vi "Append Table.vi"(0 "PDF Report IN":T30(xcontrol), 1 "Title format":T2={"Font"={"Name"="", "Size"=-1.0, "Color"=0, "Style"={"Bold"=TRUE, "Italic"=FALSE, "Underline"=FALSE, "Strikeout"=FALSE}}, "Align. and LS"={"Horizontal"=enum."CENTER", "Vertical"=enum."MIDDLE", "Line spacing"=enum."1.0"}}, 2 "Predefined Borders":T14={"Borders"=1, "Title"={"Thickness"=1.0, "Line"=0, "Background "=16777215}, "Datas"={"Thickness"=0.5, "Line"=0, "Background "=16777215}}, 3 "Row background color":T9={"color"=16777225, "at each"=0.0}, 7 "PDF Table":T1(xcontrol), 9 "Caption":string, 11 "error in (no error)":errorcluster, 12 "Datas format":T2={"Font"={"Name"="", "Size"=-1.0, "Color"=0, "Style"={"Bold"=FALSE, "Italic"=FALSE, "Underline"=FALSE, "Strikeout"=FALSE}}, "Align. and LS"={"Horizontal"=enum."CENTER", "Vertical"=enum."MIDDLE", "Line spacing"=enum."1.0"}}, 13 "Custom Borders":T13={"Title Row Border"={"Line"={"Thickness"=1.0, "Color"=0}, "Column Borders [ ]"=[]}, "Datas Row Borders [ ]"=[]}) -> (4 "PDF Report OUT":T30(xcontrol), 15 "error out":errorcluster)   [LabVIEW 2012]
doc: "<B>ENGLISH</B>\nAppends a table to the PDF document.\n\n<B>FRANÇAIS</B>\nAjoute un tableau au document PDF.\n\nDeveloped by Jean-Marc Simard\nCopyright © 2010, Exaprom Inc.\nAll rights reserved.\nLicense: BSD\n\nWith iTextSharp 4.1.6 (http://itextsharp.sourceforge.net)\nunder Mozilla Public License Version 1.1\n(http://www.mozilla.org/MPL/MPL-1.1.html)"
uses:
  Controls/PDF Report Xcontrol/PDF Report.xctl
  Controls/Row Predefined borders cluster.ctl
  Controls/Row Predefined borders.ctl
  Controls/Row Border Title.ctl
  Controls/Cell Border.ctl
  Controls/Row Borders [ ] Datas.ctl
  Controls/Row Back Ground color Datas.ctl
  Controls/Cell Properties Table.ctl
  Controls/Font cluster.ctl
  Controls/Font size.ctl
  Controls/Font color.ctl
  Controls/Texte alignement.ctl
  Controls/Cell Vertical alignment.ctl
  Controls/Line spacing.ctl
  Controls/PDF Table Xcontrol/PDF Table XControl.xctl
  Controls/Row borders from.ctl
  C:/Users/MaxCorp/Documents/TopPerm - Base/DLL/itextsharp.dll
  DLL/itextsharp.dll
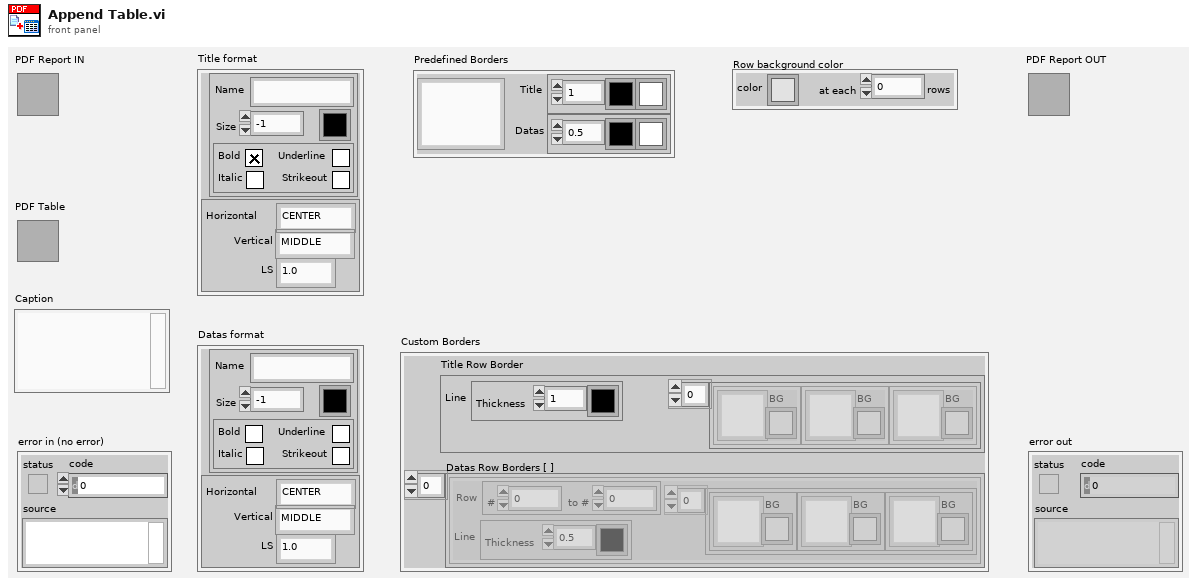
[diagram p1: front panel]
types:
  T1 = cluster{"PDFTable ref":refnum<k24>, "columnWidth (points)":sgl[], "Title 1D":string[], "Table Datas 2D":string[][], "Image to Add with refnum[ ]":cluster{"Image name":string, "InstanceImage":refnum<k24>}[]}
  T2 = typedef "Cell Properties Table.ctl" = cluster{"Font":T3, "Align. and LS":cluster{"Horizontal":T6, "Vertical":T7, "Line spacing":T8}}
  T3 = typedef "Font cluster.ctl" = cluster{"Name":string, "Size":T4, "Color":T5, "Style":cluster{"Bold":bool, "Italic":bool, "Underline":bool, "Strikeout":bool}}
  T4 = typedef "Font size.ctl" = sgl
  T5 = typedef "Font color.ctl" = u32
  T6 = typedef "Texte alignement.ctl" = enum16{"Select", "CENTER", "JUSTIFY", "LEFT", "RIGHT"}
  T7 = typedef "Cell Vertical alignment.ctl" = enum16{"TOP", "MIDDLE", "BOTTOM"}
  T8 = typedef "Line spacing.ctl" = enum16{"Select", "1.0", "1.5", "2.0"}
  T9 = typedef "Row Back Ground color Datas.ctl" = cluster{"color":u32, "at each":dbl}
  T10 = typedef "Row Border Title.ctl" = cluster{"Line":cluster{"Thickness":sgl, "Color":u32}, "Column Borders [ ]":cluster{"Cell Border":T11, "BG":u32}[]}
  T11 = typedef "Cell Border.ctl" = u16
  T12 = typedef "Row Borders [ ] Datas.ctl" = cluster{"Row":cluster{"#":i16, "to #":i16}, "Line":cluster{"Thickness":sgl, "Color":u32}, "Column Borders [ ]":cluster{"Cell Border":T11, "BG":u32}[]}[]
  T13 = cluster{"Title Row Border":T10, "Datas Row Borders [ ]":T12}
  T14 = typedef "Row Predefined borders cluster.ctl" = cluster{"Borders":T15, "Title":cluster{"Thickness":sgl, "Line":u32, "Background ":u32}, "Datas":cluster{"Thickness":sgl, "Line":u32, "Background ":u32}}
  T15 = typedef "Row Predefined borders.ctl" = u16
  T16 = typedef "Unit.ctl" = enum16{"inch", "mm"}
  T17 = typedef "Paragraphe cluster.ctl" = cluster{" Aligment":T6, "Line spacing":T8}
  T18 = typedef "Page dimensions.ctl" = cluster{"Start at page":i32, "Orientation":T19, "widht":sgl, "height":sgl, "Margin left":sgl, "Margin right":sgl, "Margin top":sgl, "Margin bottom":sgl}
  T19 = typedef "Page Orientation.ctl" = enum16{"Portrait", "Landscape"}
  T20 = typedef "Image or Table Caption.ctl" = cluster{"Caption":string, "Separator":string, "Position":enum16{"Above", "Below"}}
  T21 = typedef "Header Footer [ ].ctl" = T22[]
  T22 = typedef "Header Footer cluster.ctl" = cluster{"Start page":i32, "Type":T23, "Alignment":T24, "Vertical Alignement":T7, "Image (%)":sgl, "Page #":T25, "Text":string, "Path":string, "Font":T3, "Font refnum":refnum<k24>, "Line":cluster{"Line":T26, "Thickness (points)":sgl, "Colour":T5}}
  T23 = typedef "Header Footer Type.ctl" = enum16{"Select", "Text", "Text + hyperlink", "Page number", "Image", "Image + hyperlink"}
  T24 = typedef "Header footer horiz alignment.ctl" = enum16{"Left", "Center", "Right"}
  T25 = typedef "Page number.ctl" = cluster{"Text 1":string, "Text 2":string, "Text 3":string}
  T26 = typedef "Header Footer Line.ctl" = enum16{"No line", "Horizontal line"}
  T27 = typedef "Watermark cluster2.ctl" = cluster{"Show? (F)":bool, "Type":enum16{"Image", "Text"}, "Opacity (%)":sgl, "Rotate(°)":sgl, "Position":cluster{"Position":T28, "X":sgl, "Y":sgl}, "Image path":path, "Scaled(%)":sgl, "Image refnum":refnum<k24>, "Text":string, "Font":cluster{"Name":string, "Size":T4, "Color":T5}, "Font refnum":refnum<k24>, "Alignment":T24, "Automatic":bool}
  T28 = typedef "Watermark Position.ctl" = enum16{"Absolute", "Center (page)", "Center (text section)"}
  T29 = typedef "System Fonts.ctl" = cluster{"Font name [ ]":string[], "Font and file names [ ]":cluster{"Font name":string, "File name":string}[]}
  T30 = cluster{"Document":refnum<k24>, "Writer":refnum<k24>, "Default Font":refnum<k24>, "Default Font cluster":T3, "Path":path, "Unit (default = mm)":T16, "Paragraphe cluster":T17, "Pages dimensions [ ]":T18[], "Captions":cluster{"Image":T20, "Image counter":u16, "Table":T20, "Table counter":u16, "Font":T3}, "Header":T21, "Footer":T21, "Watermark ":T27, "Actual VI name":string, "System Fonts":T29}
  T31 = typedef "Row borders from.ctl" = enum16{"Title", "Datas"}
  T32 = cluster{"Image name":string, "InstanceImage":refnum<k24>}[]
  T33 = typedef "Cell Generic Format without Font.ctl" = cluster{"Font Ref":refnum<k24>, "Line":cluster{"Thickness":sgl, "Color":u32}, "Borders and BG":cluster{"Cell Border":T11, "BG":u32}, "PdfPCell refnum":refnum<k24>}
  T34 = cluster{"Cell [ ]":T33[], "Close Font Ref":cluster{"Title":bool, "Title Font Ref":refnum<k24>, "Datas":bool, "Data Font Ref":refnum<k24>}}
  T35 = typedef "Row PdfPCell [ ] Datas.ctl" = cluster{"Row":cluster{"#":i16, "to #":i16}, "Cell Cluster":T36, "PdfPCell [ ]":refnum<k24>[]}[]
  T36 = typedef "Cell Cluster.ctl" = cluster{"Font Ref":refnum<k24>, "Leading":T4, "Horizontal Aligment":T6, "Vertical Alignment":T7}
  T37 = typedef "Title Cells with refnum.ctl" = cluster{"Cell Cluster":T36, "PdfPCell [ ]":refnum<k24>[]}
  T38 = cluster{"Row":cluster{"#":i16, "to #":i16}, "Cell Cluster":T36, "PdfPCell [ ]":refnum<k24>[]}
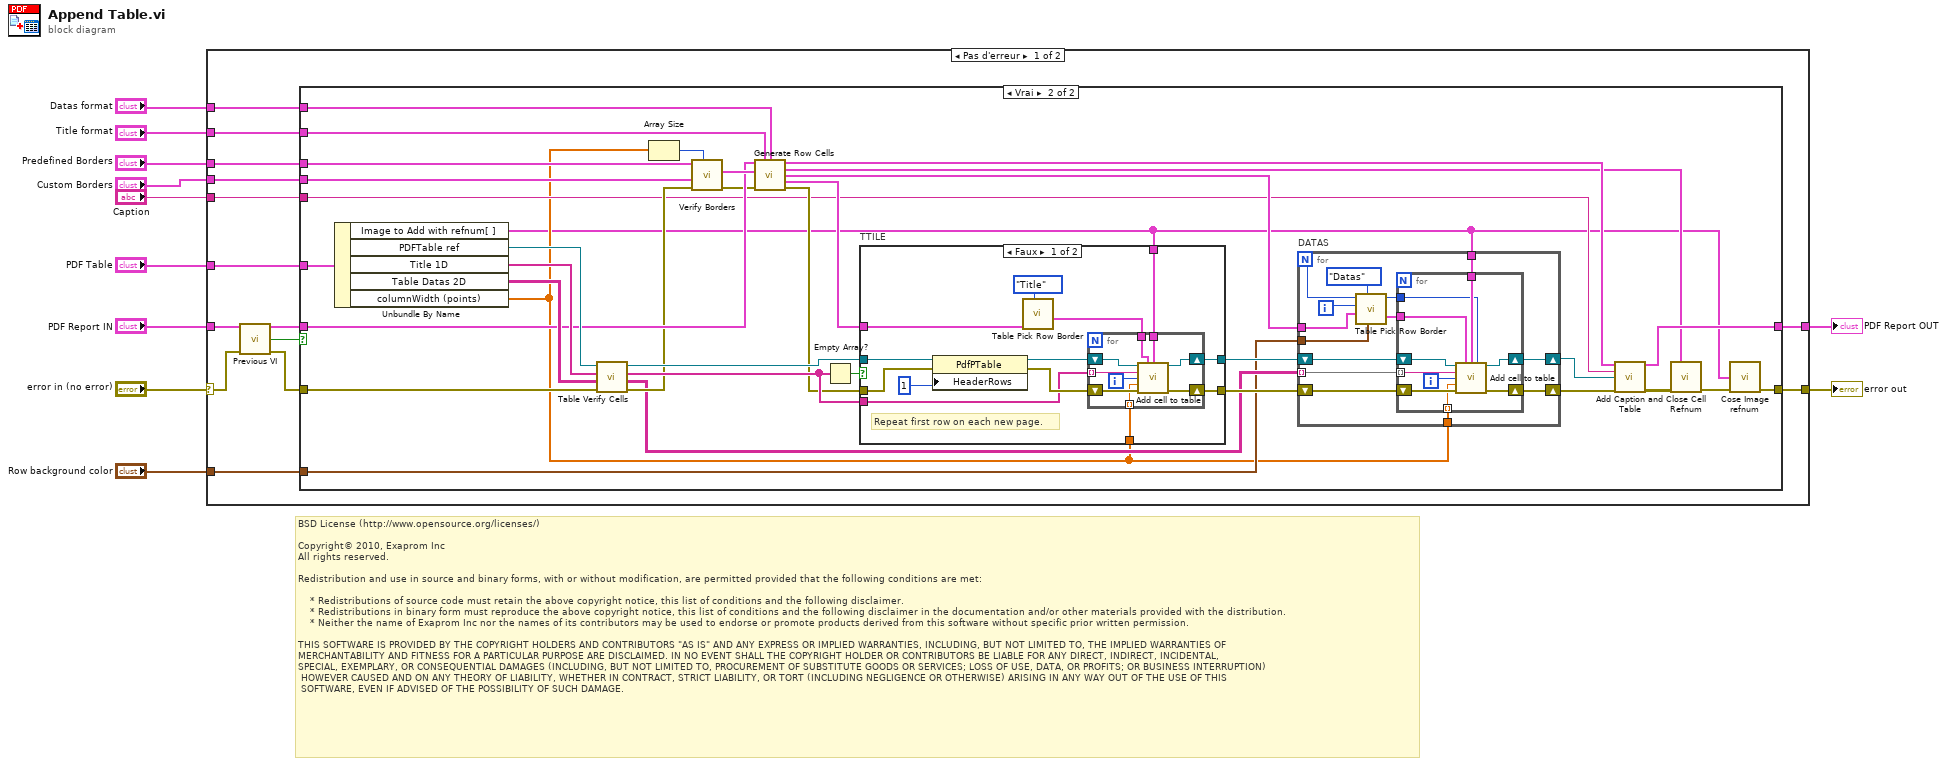
[diagram p0: block diagram]
diagram:
  # "BSD License (http://www.opensource.org/licenses/)\n\nCopyright© 2010, Exaprom Inc\nAll rights reserved.\n\nRedistribution and use in source and binary forms, with or without modification, are permitted provided that the following conditions are met:\n\n    * Redistributions of source code must retain the above copyright notice, this list of conditions and the following disclaimer.\n    * Redistributions in binary form must reproduce the above copyright notice, this list of conditions and the following disclaimer in the documentation and/or other materials provided with the distribution.\n    * Neither the name of Exaprom Inc nor the names of its contributors may be used to endorse or promote products derived from this software without specific prior written permission.\n\nTHIS SOFTWARE IS PROVIDED BY THE COPYRIGHT HOLDERS AND CONTRIBUTORS \"AS IS\" AND ANY EXPRESS OR IMPLIED WARRANTIES, INCLUDING, BUT NOT LIMITED TO, THE IMPLIED WARRANTIES OF \nMERCHANTABILITY AND FITNESS FOR A PARTICULAR PURPOSE ARE DISCLAIMED. IN NO EVENT SHALL THE COPYRIGHT HOLDER OR CONTRIBUTORS BE LIABLE FOR ANY DIRECT, INDIRECT, INCIDENTAL,\nSPECIAL, EXEMPLARY, OR CONSEQUENTIAL DAMAGES (INCLUDING, BUT NOT LIMITED TO, PROCUREMENT OF SUBSTITUTE GOODS OR SERVICES; LOSS OF USE, DATA, OR PROFITS; OR BUSINESS INTERRUPTION)\n HOWEVER CAUSED AND ON ANY THEORY OF LIABILITY, WHETHER IN CONTRACT, STRICT LIABILITY, OR TORT (INCLUDING NEGLIGENCE OR OTHERWISE) ARISING IN ANY WAY OUT OF THE USE OF THIS\n SOFTWARE, EVEN IF ADVISED OF THE POSSIBILITY OF SUCH DAMAGE."
  n1 = case shown="Pas d'erreur" "error in (no error)" {
    selector: "error in (no error)" -> [w13 w112]
    tunnel: [w23 w112] -> w1
    tunnel: "PDF Report IN" -> [w20 w111]
    tunnel: [w25 w111] -> w9
    tunnel: "Title format" -> [w21 _]
    tunnel: "Datas format" -> [w19 _]
    tunnel: "Caption" -> [w24 _]
    tunnel: "PDF Table" -> [w22 _]
    tunnel: "Predefined Borders" -> [w18 _]
    tunnel: "Custom Borders" -> [w17 _]
    tunnel: "Row background color" -> [w16 _]
    frame No Error {
      n2 = call "Previous VI.vi"("PDF Report IN"=w20, "error in (no error)"=w13) -> ("PDF Report OUT"=w15:T30, "Execute Actual VI"=w14:bool, "error out"=w12:errorcluster)  [unwired: 11 out]
      n3 = case shown="Vrai" w14 {
        tunnel: [w27 w40] -> w25
        tunnel: w24 -> [_ w35]
        tunnel: [w26 w29] -> w23
        tunnel: w22 -> [_ w59]
        tunnel: w21 -> [_ w52]
        tunnel: w19 -> [_ w50]
        tunnel: w12 -> [w26 w58]
        tunnel: w18 -> [_ w54]
        tunnel: w17 -> [_ w53]
        tunnel: w16 -> [_ w33]
        tunnel: w15 -> [w27 w48]
        frame False {
        }
        frame True {
          n4 = Unbundle By Name(w59) -> ("Image to Add with refnum[ ]"=w28:T32, "PDFTable ref"=w57:refnum<k24>, "Title 1D"=w56:string[], "Table Datas 2D"=w55:string[][], "columnWidth (points)"=w32:sgl[])
          n5 = call "Table Verify Cells.vi"("error in (no error)"=w58, "Table Datas 2D IN"=w55, "Title 1D IN"=w56, "PdfP Table"=w57) -> ("error out"=w46:errorcluster, "Table Datas 2D OUT"=w34:string[][], "Title 1D OUT"=w60:string[], "PdfP Table duplicate"=w61:refnum<k24>)  [unwired: 4 out]
          n6 = Array Size(array=w32) -> (size(s)=w36:i32)
          n7 = call "Verify Borders.vi"("Column Number"=w36, "error in (no error)"=w46, "Borders IN"=w53, "Predefined Borders"=w54) -> ("error out"=w47:errorcluster, "Borders OUT"=w49:T13)  [unwired: 6 out]
          n8 = call "Generate Row Cells.vi"("PDF Report"=w48, "Title format"=w52, "Datas format"=w50, "Custom Borders"=w49, "error in (no error)"=w47) -> ("PDF Report duplicate"=w42:T30, "References"=w37:T34, "Datas Row Cells [ ]"=w43:T35, "Title Row Cells"=w44:T37, "error out"=w45:errorcluster)  [unwired: 2 in, 4 out]
          n9 = Empty Array?(array=w60) -> (empty?=w31:bool)
          n10 = case "TTILE" shown="Faux" w31 {
            tunnel: [w97 w110] -> w62
            tunnel: [w96 w109] -> w51
            tunnel: w61 -> [w95 w110]
            tunnel: w45 -> [w99 w109]
            tunnel: w60 -> [w94 _]
            tunnel: w28 -> [w91 _]
            tunnel: w32 -> [w90 _]
            tunnel: w44 -> [w87 _]
            frame False {
              # "Repeat first row on each new page."
              n11 = property class="PdfPTable"(reference=w95, error in=w99, "HeaderRows"=1) -> (reference out=w93:refnum<k24>, error out=w98:errorcluster)
              n12 = call "Table Pick Row Border.vi"("Row borders from"=Row_borders_from."Title", "Title Row Cells"=w87) -> ("Row Borders"=w89:T38)  [unwired: 4 in, 5 out]
              n13 = for {
                shift-right: [w108] -> w97
                shift-left: w93 -> [w106]
                shift-right: [w107] -> w96
                shift-left: w98 -> [w105]
                tunnel: w94 -> [w104] mode=indexing
                tunnel: w91 -> [w103]
                tunnel: w90 -> [w102] mode=indexing
                tunnel: w89 -> [w101]
                i -> [w100]
                n14 = call "Add cell to table.vi"("PdfP Table"=w106, "Row Borders"=w101, "Image to Add [ ]"=w103, "String"=w104, "i"=w100, "Column Width (points)"=w102, "error in (no error)"=w105) -> ("PdfP Table duplicate"=w108:refnum<k24>, "error out"=w107:errorcluster)  [unwired: 2 in, 5 out]
              }
            }
            frame True {
            }
          }
          n15 = for "DATAS" {
            N -> [w69]
            shift-right: [w76] -> w41
            shift-left: w62 -> [w74]
            shift-right: [w75] -> w39
            shift-left: w51 -> [w73]
            tunnel: w34 -> [w72] mode=indexing
            tunnel: w28 -> [w71]
            tunnel: w32 -> [w70]
            tunnel: w43 -> [w66]
            tunnel: w33 -> [w65]
            i -> [w67]
            n16 = call "Table Pick Row Border.vi"("Data Row Back Ground color"=w65, "Row borders from"=Row_borders_from."Datas", "Datas Row Cells [ ]"=w66, "i"=w67, "N"=w69) -> ("Row Borders"=w68:T38, "Background Color"=w64:u32)  [unwired: 1 in, 4 out]
            n17 = for {
              shift-right: [w86] -> w76
              shift-left: w74 -> [w84]
              shift-right: [w85] -> w75
              shift-left: w73 -> [w83]
              tunnel: w72 -> [w82] mode=indexing
              tunnel: w71 -> [w81]
              tunnel: w70 -> [w80] mode=indexing
              tunnel: w68 -> [w78]
              tunnel: w64 -> [w77]
              i -> [w79]
              n18 = call "Add cell to table.vi"("PdfP Table"=w84, "Row Borders"=w78, "Image to Add [ ]"=w81, "Back Ground Color"=w77, "String"=w82, "i"=w79, "Column Width (points)"=w80, "error in (no error)"=w83) -> ("PdfP Table duplicate"=w86:refnum<k24>, "error out"=w85:errorcluster)  [unwired: 1 in, 5 out]
            }
          }
          n19 = call "Add Caption and Table.vi"("PDF Report IN"=w42, "Caption"=w35, "PdfPTable"=w41, "error in (no error)"=w39) -> ("PDF Report OUT"=w40:T30, "error out"=w38:errorcluster)  [unwired: 10 out]
          n20 = call "Close Cell Refnum.vi"("References"=w37, "error in (no error)"=w38) -> ("error out"=w30:errorcluster)  [unwired: 2 in, 11 out]
          n21 = call "Cose Image refnum.vi"("Image to Add refnum [ ]"=w28, "error in (no error)"=w30) -> ("error out"=w29:errorcluster)  [unwired: 13 out]
        }
      }
    }
    frame Error {
    }
  }
  "error out" <- w1
  "PDF Report OUT" <- w9
